vi "H5Lget_val (Basic).vi"(6 "lapl_id":T2, 8 "error in (no error)":errorcluster, 10 "Name":string=".", 11 "Location Ref":T2) -> (0 "error out":errorcluster, 1 "buffer":u8[](array[numeric]), 3 "Location Ref out":T2, 4 "type":T1 items=["H5L_TYPE_ERROR"=-1, "H5L_TYPE_HARD"=0, "H5L_TYPE_SOFT"=1, "H5L_TYPE_EXTERNAL"=64, "H5L_TYPE_MAX"=255])   [LabVIEW 2017]
doc: "Returns the value of a symbolic link."
uses:
  <vilib>/UPVI/lvhdf5/library.llb/HDF5 Ref.ctl
  <vilib>/UPVI/lvhdf5/link.llb/H5L_type_t.ctl
  <vilib>/UPVI/lvhdf5/error.llb/LVH5EMajorID.ctl
  <vilib>/UPVI/lvhdf5/error.llb/LVH5EMinorID.ctl
  <vilib>/UPVI/lvhdf5/error.llb/H5Epush_enum_enum.vi
  <vilib>/UPVI/lvhdf5/hdf5.dll
panel:
  # "LVHDF5 Toolkit\nCopyright (c) 2005-2013 by Jason D. Sommerville\nCopyright (c) 2014-2015 by UPVI, LLC.\n\nThis use and distribution of this file is governed by the terms found in \nLICENSE.txt distributed with this toolkit and installed at\n <user.lib>\\_lvhdf5\\LICENSE.txt"
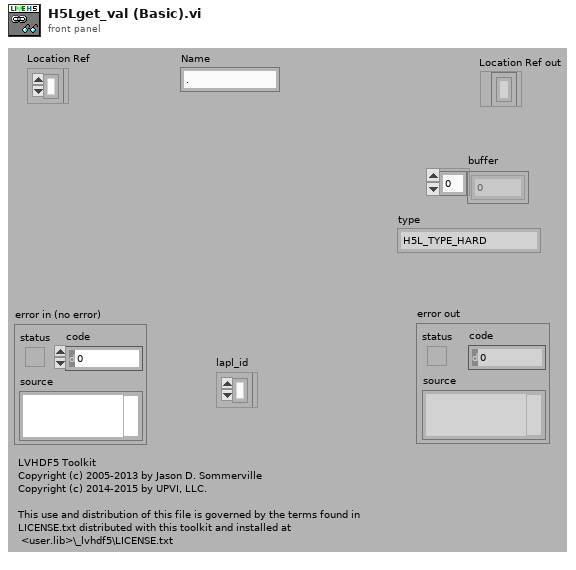
[diagram p1: front panel]
types:
  T1 = typedef "H5L_type_t.ctl" = i32
  T2 = typedef "HDF5 Ref.ctl" = refnum<k1>
  T3 = typedef "LVH5EMinorID.ctl" = string
  T4 = typedef "LVH5EMajorID.ctl" = string
  T5 = typedef "H5L_info_t.ctl" = cluster{"type":T1, "corder_valid":bool, "corder":i64, "cset":T6, "address/val_size":u64}
  T6 = typedef "H5T_cset_t.ctl" = i32
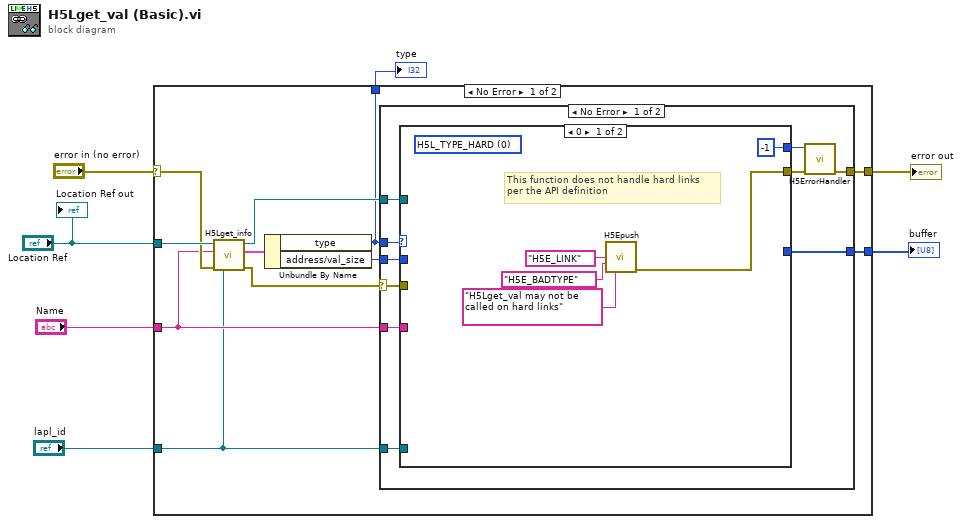
[diagram p0: block diagram]
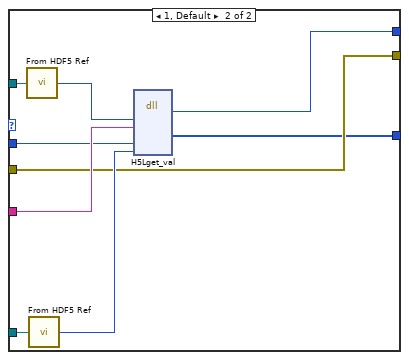
[diagram p2: hidden frame]
diagram:
  n1 = case shown="No Error" "error in (no error)" {
    selector: "error in (no error)" -> [w16 w43]
    tunnel: [w18 w43] -> w6
    tunnel: "lapl_id" -> [w8 _]
    tunnel: "Location Ref" -> [w17 _]
    tunnel: "Name" -> [w11 _]
    tunnel: [w10 _] -> w2
    tunnel: [w9 _] -> w1
    frame No Error {
      n2 = call <vilib>:"H5Lget_info.vi"("lapl_id"=w8, "error in (no error)"=w16, "Name"=w11, "Location Ref"=w17) -> ("error out"=w14:errorcluster, "H5L_info_t"=w15:T5, "Location Ref out"=w13:T2)  [unwired: 5 in]
      n3 = Unbundle By Name(w15) -> ("type"=w9:T1, "address/val_size"=w12:u64)
      n4 = case shown="No Error" w14 {
        selector: w14 -> [w23 w42]
        tunnel: [w27 w42] -> w18
        tunnel: w9 -> [w26 _]
        tunnel: w13 -> [w25 _]
        tunnel: w12 -> [w24 _]
        tunnel: w11 -> [w22 _]
        tunnel: w8 -> [w21 _]
        tunnel: [w19 _] -> w10
        frame No Error {
          n5 = case shown="0" w26 {
            tunnel: [w29 w34] -> w27
            tunnel: w25 -> [_ w41]
            tunnel: w24 -> [_ w38]
            tunnel: w23 -> [_ w34]
            tunnel: w22 -> [_ w39]
            tunnel: w21 -> [_ w37]
            tunnel: [-1 ("return type") w35] -> w20
            tunnel: [_ w33] -> w19
            frame 0 {
              (unwired) T1 0 items=["H5L_TYPE_ERROR"=-1, "H5L_TYPE_HARD"=0, "H5L_TYPE_SOFT"=1, "H5L_TYPE_EXTERNAL"=64, "H5L_TYPE_MAX"=255] ("type")
              # "This function does not handle hard links\nper the API definition"
              n6 = call-poly <vilib>:"H5Epush.vi"("major_id"=T4 "H5E_LINK", "minor_id"=T3 "H5E_BADTYPE", "msg"="H5Lget_val may not be called on hard links") -> ("error out"=w29:errorcluster)  [unwired: 11 in, 1 out]
            }
            frame 1, Default {
              n7 = call <vilib>:"From HDF5 Ref.vi"("HDF5 Ref"=w41) -> ("I32"=w40:i32)
              n8 = call <vilib>:"From HDF5 Ref.vi"("HDF5 Ref"=w37) -> ("I32"=w36:i32)
              n9 = dll-call lib="C:/Program Files/National Instruments/LabVIEW 2017/vi.lib/UPVI/lvhdf5/hdf5.dll" fn="H5Lget_val"("loc_id"=w40, "name"=w39, "size"=w38, "lapl_id"=w36) -> ("return type"=w35:i32, "buff"=w33:u8[])  [unwired: 8 in, 2 out]
            }
          }
          n10 = call <vilib>:"H5ErrorHandler.vi"("herr_t"=w20) -> ()  [unwired: 4 in, 5 out]
        }
        frame Error {
        }
      }
    }
    frame Error {
    }
  }
  "error out" <- w6
  "buffer" <- w2
  "type" <- w1
  "Location Ref out" <- "Location Ref"
